vi "Class to Main_to_gRPC.vi"(11 "Timed Node in":refnum<class "AMS Chiller Template.lvclass">) -> (2 "Main to gRPC":T1, 3 "Timed Node out":refnum<class "AMS Chiller Template.lvclass">)   [LabVIEW 2023, in "AMS Chiller Template.lvlib" / "AMS Chiller Template.lvclass"]
uses:
  AMS Chiller Template.lvclass
  Type Defs/Main to gRPC.ctl
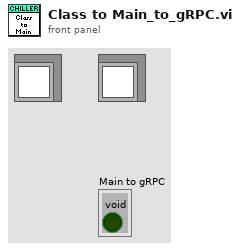
[diagram p1: front panel]
types:
  T1 = typedef "AMS Chiller Template.lvlib/AMS Chiller Template.lvclass/Main to gRPC.ctl" = cluster{"void":bool}
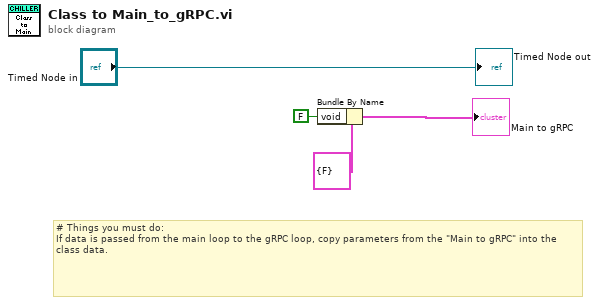
[diagram p0: block diagram]
diagram:
  # "# Things you must do:\nIf data is passed from the main loop to the gRPC loop, copy parameters from the \"Main to gRPC\" into the class data."
  n1 = Bundle By Name(cluster=T1 {"void"=FALSE} ("Main to gRPC"), "void"=FALSE) -> (→"Main to gRPC":T1)
  "Timed Node out" <- "Timed Node in"
